vi "Write Tag Name.vi"(8 "error in (no error)":errorcluster, 10 "Tag Name":string, 11 "Update Tag in":refnum<class "Update Tag.lvclass">) -> (0 "error out":errorcluster, 3 "Update Tag out":refnum<class "Update Tag.lvclass">)   [LabVIEW 2018, in "Update Tag.lvclass"]
uses:
  Update Tag.lvclass
  Update Tag.lvclass/Update Tag.ctl
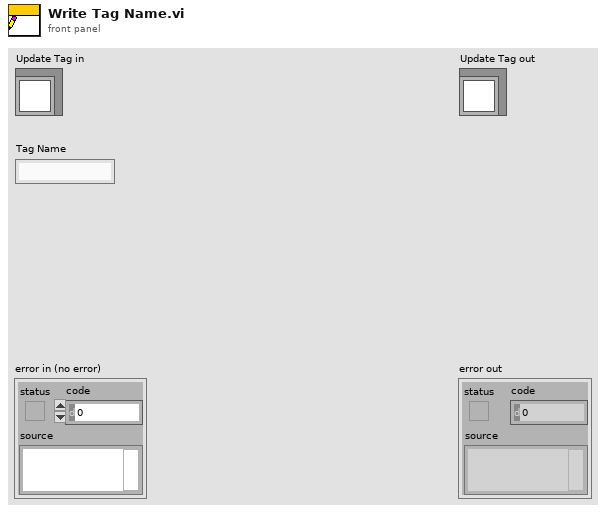
[diagram p1: front panel]
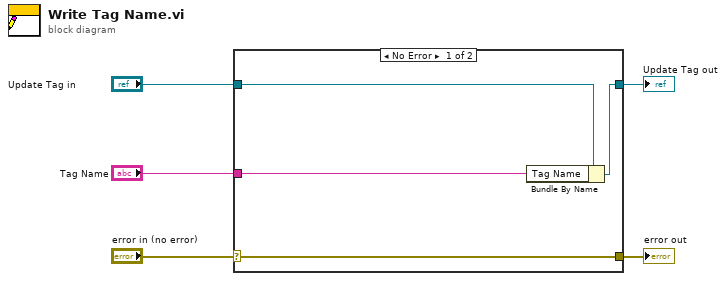
[diagram p0: block diagram]
diagram:
  n1 = case shown="No Error" "error in (no error)" {
    selector: "error in (no error)" -> [w9 w10]
    tunnel: [w9 w10] -> w4
    tunnel: [w7 w11] -> w2
    tunnel: "Update Tag in" -> [w8 w11]
    tunnel: "Tag Name" -> [w6 _]
    frame No Error {
      n2 = Bundle By Name(cluster=w8, "Tag Name"=w6) -> (w7:refnum<class "Update Tag.lvclass">)
    }
    frame Error {
    }
  }
  "error out" <- w4
  "Update Tag out" <- w2
